vi "select current channel.vi"(10 "Current Motion":T3, 11 "Motor Type":T1) -> (3 "Analog channel":T2)   [LabVIEW 2018]
uses:
  02.Type Def's/All Motions.ctl
  02.Type Def's/EOL Analog Input Control.ctl
  05.UserVI's/type defs/EOL Motor Type.ctl
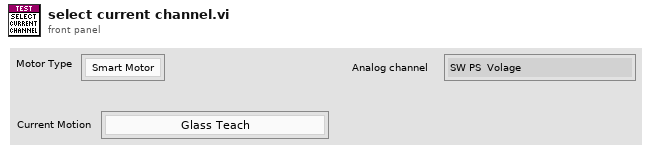
[diagram p1: front panel]
types:
  T1 = typedef "EOL Motor Type.ctl" = enum16{"Smart Motor", "Sensor Motor"}
  T2 = typedef "EOL Analog Input Control.ctl" = enum16{"SW PS  Volage", "Switch A", "Switch B", "Switch C", "Motor Voltage", "Motor Current", "ATS"}
  T3 = typedef "All Motions.ctl" = enum16{"Glass Teach", "Glass Slide Open", "Glass Slide Close", "Glass Vent Open", "Glass Vent Close", "Sunshade Teach", "Sunshade Open", "Sunshade Close", "Idle", "Sunshade Open 2", "Sunshade Close 2", "Glass Slide Open Sunshade Open", "Glass Slide Open Sunshade Close", "Glass Slide Close Sunshade Open", "Glass Slide Close Sunshade Close", "Glass Vent Open Sunshade Open", "Glass Vent Open Sunshade Close", "Glass Vent Close Sunshade Open", "Glass Vent Close Sunshade Close", "Express Glass Slide Open", "Express Glass Slide Close", "Express Glass Vent Open", "Express Glass Vent Close", "Express Sunshade Open", "Express Sunshade Close", "Express Sunshade Open 2", "Express Sunshade Close 2", "Express Glass Slide Open Sunshade Open", "Express Glass Slide Open Sunshade Close", "Express Glass Slide Close Sunshade Open", "Express Glass Slide Close Sunshade Close", "Express Glass Vent Open Sunshade Open", "Express Glass Vent Open Sunshade Close", "Express Glass Vent Close Sunshade Open", "Express Glass Vent Close Sunshade Close", "Goto Position Glass", "Goto Position Sunshade", "Sunshade Teach 2"}
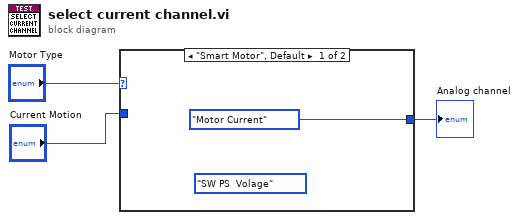
[diagram p0: block diagram]
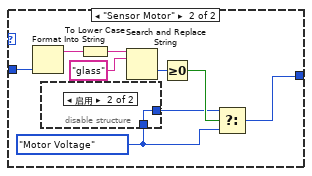
[diagram p2: hidden frame]
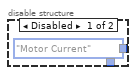
[diagram p3: hidden frame]
diagram:
  n1 = case shown="\"Smart Motor\", Default" "Motor Type" {
    tunnel: [EOL_Analog_Input_Control."Motor Current" ("Analog Control") w6] -> w2
    tunnel: "Current Motion" -> [_ w13]
    frame "Smart Motor", Default {
      (unwired) EOL_Analog_Input_Control."SW PS  Volage" ("Analog Control")
    }
    frame "Sensor Motor" {
      w5 = EOL_Analog_Input_Control."Motor Voltage" ("Analog Control")
      n2 = Format Into String(w13) -> (resulting string=w12:string)  [unwired: 3 in, 1 out]
      n3 = disable-structure shown="启用" {
        disable-tunnel: [EOL_Analog_Input_Control."Motor Current" ("Analog Control") w15] -> w7
        disable-tunnel: w5 -> [_ w15]
        frame Disabled {
        }
        frame Enabled {
        }
      }
      n4 = To Lower Case(string=w12) -> (all lower case string=w11:string)
      n5 = Search and Replace String(input string=w11, search string="glass") -> (offset past replacement=w9:i32)  [unwired: 6 in, 3 out]
      n6 = Greater Or Equal To 0?(x=w9) -> (x >= 0?=w8:bool)
      n7 = Select(t=w7, s=w8, f=w5) -> (s? t:f=w6:T2)
    }
  }
  "Analog channel" <- w2
